vi "RemoveTimeInfo.vi"(9 "Error in":errorcluster) -> (1 "Error out":errorcluster, 4 "Removed time info":string)   [LabVIEW 2017, in "GPError.lvlib"]
doc: "Removes time info from the source string of <B>Error in</B> and returns the modified error cluster in <B>Error out</B>. If any time info is found it is returned in <B>Removed time info</B>.\n\nNote that this VI is not intended for use on appended errors!\n\nThis VI is inlined.\n\nSteen Schmidt\nGPower\n10/7 2013"
uses:
  GPError.lvlib
panel:
  # "Copyright © 2013\nSteen Schmidt, GPower\nSee enclosed license file for terms and conditions"
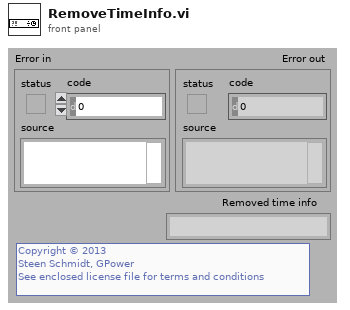
[diagram p1: front panel]
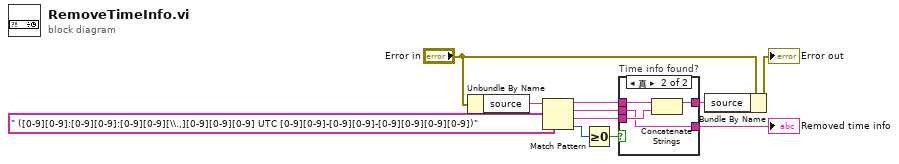
[diagram p0: block diagram]
diagram:
  n1 = Unbundle By Name("Error in") -> ("source"=w11:string)
  n2 = Match Pattern(string=w11, regular expression=" ([0-9][0-9]:[0-9][0-9]:[0-9][0-9][\\.,][0-9][0-9][0-9] UTC [0-9][0-9]-[0-9][0-9]-[0-9][0-9][0-9][0-9])" ("time format string (%c)")) -> (before substring=w5:string, match substring=w6:string, after substring=w7:string, offset past match=w9:i32)  [unwired: 1 in]
  n3 = Greater Or Equal To 0?(x=w9) -> (x >= 0?=w8:bool)
  n4 = case "Time info found?" shown="真" w8 {
    tunnel: w7 -> [_ w15]
    tunnel: w6 -> [_ w13]
    tunnel: w5 -> [w12 w16]
    tunnel: [w12 w14] -> w3
    tunnel: [_ w13] -> w1
    frame False {
    }
    frame True {
      n5 = Concatenate Strings(w16, w15) -> (w14:string)
    }
  }
  "Removed time info" <- w1
  n6 = Bundle By Name(cluster="Error in", "source"=w3) -> (→"Error out":errorcluster)
